vi "Analyse.vi"(8 "error in (no error)":errorcluster, 11 "ResultHandler JSON in":refnum<class "ResultHandler JSON.lvclass">) -> (0 "error out":errorcluster, 1 "ICallResult":refnum<class "ICallResult.lvclass">, 2 "Request ID":u64, 3 "ResultHandler JSON out":refnum<class "ResultHandler JSON.lvclass">)   [LabVIEW 2020, in "wamplv.lvlib" / "ResultHandler JSON.lvclass"]
uses:
  ResultHandler JSON.lvclass
  ResultHandler JSON.lvclass/ResultHandler JSON.ctl
  <vilib>/Utility/error.llb/Error Cluster From Error Code.vi
  <vilib>/ErrorRing/Error Ring.xnode
  Error/ErrorHandler JSON/ErrorHandler JSON.lvclass
  SerialisedMessages/JSONMessage/WampMessage JSON.lvclass
  Call/CallResult JSON/CallResult JSON.lvclass
  Utils/Utils.lvclass
  Call/ICallResult/ICallResult.lvclass
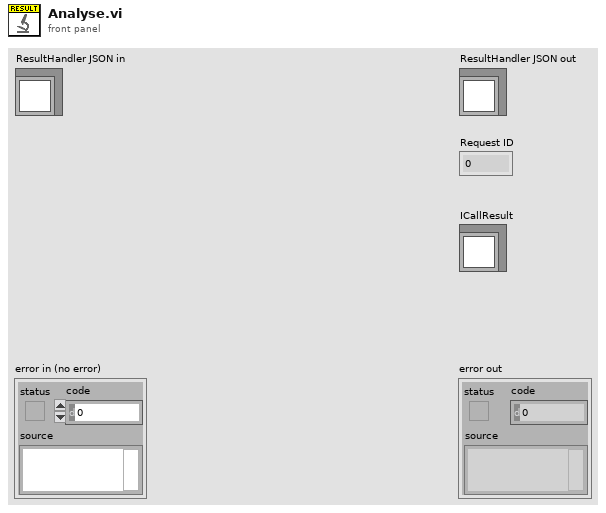
[diagram p1: front panel]
types:
  T1 = typedef "wamplv.lvlib/WAMP Message Codes.ctl" = enum8{"HELLO", "WELCOME", "CHALLENGE", "AUTHENTICATE", "ABORT", "GOODBYE", "ERROR", "PUBLISH", "PUBLISHED", "SUBSCRIBE", "SUBSCRIBED", "UNSUBSCRIBE", "UNSUBSCRIBED", "EVENT", "CALL", "RESULT", "REGISTER", "REGISTERED", "UNREGISTER", "UNREGISTERED", "INVOCATION", "YIELD"}
  T2 = typedef "wamplv.lvlib/Error (JSON).ctl" = cluster{"Request ID":u64, "Message type that caused error":T1, "Error/Abort details (JSON)":T3}
  T3 = typedef "wamplv.lvlib/Error or abort detail (JSON).ctl" = cluster{"Error URI":string, "Error Arguments":string, "Error ArgumentKw":string, "Error Details":string, "Associated LabVIEW Error":errorcluster}
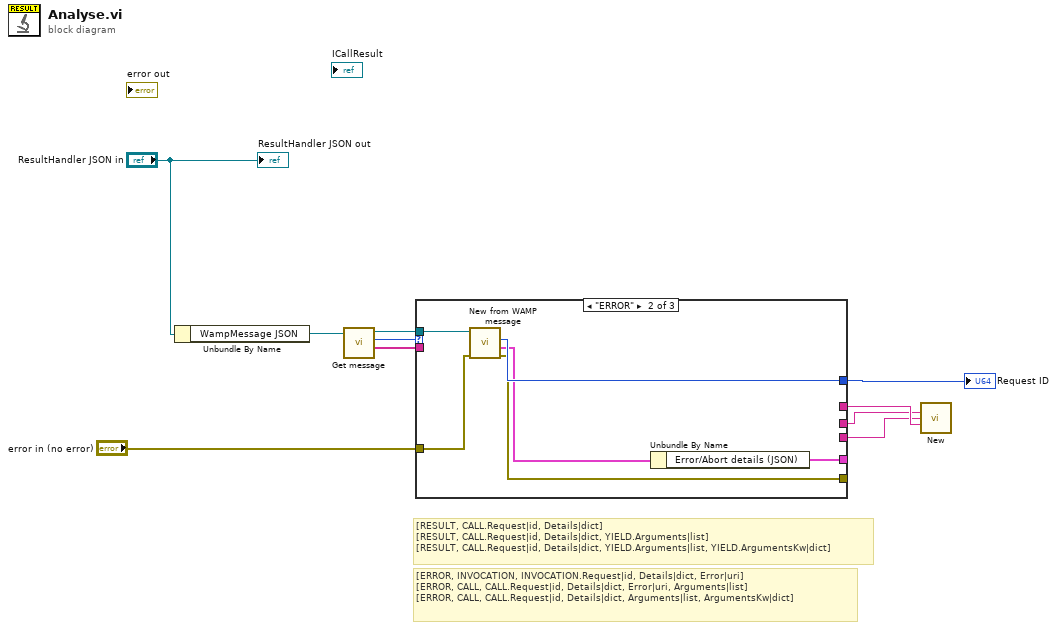
[diagram p0: block diagram]
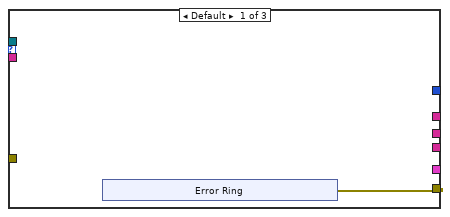
[diagram p2: hidden frame]
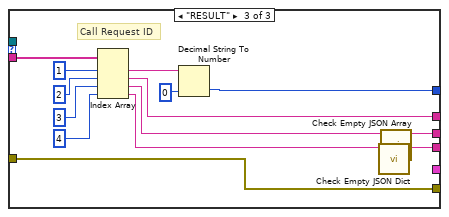
[diagram p3: hidden frame]
diagram:
  # "[RESULT, CALL.Request|id, Details|dict]\n[RESULT, CALL.Request|id, Details|dict, YIELD.Arguments|list]\n[RESULT, CALL.Request|id, Details|dict, YIELD.Arguments|list, YIELD.ArgumentsKw|dict]"
  # "[ERROR, INVOCATION, INVOCATION.Request|id, Details|dict, Error|uri]\n[ERROR, CALL, CALL.Request|id, Details|dict, Error|uri, Arguments|list]\n[ERROR, CALL, CALL.Request|id, Details|dict, Arguments|list, ArgumentsKw|dict]"
  n1 = Unbundle By Name("ResultHandler JSON in") -> ("WampMessage JSON"=w8:refnum<class "WampMessage JSON.lvclass">)
  n2 = call "Get message.vi"("JSONMessage in"=w8) -> ("<JSON>Elements"=w5:string[], "Message Type"=w7:T1, "JSONMessage out"=w6:refnum<class "WampMessage JSON.lvclass">)  [unwired: 8 in]
  n3 = case shown="\"ERROR\"" w7 {
    tunnel: [_ w18 w33] -> w4
    tunnel: [w11 w17 w32] -> _
    tunnel: [_ _ w22] -> w1
    tunnel: "error in (no error)" -> [_ w19 w32]
    tunnel: [_ w21 _] -> _
    tunnel: [_ _ w28] -> w3
    tunnel: [_ _ w24] -> w2
    tunnel: w6 -> [_ w20 _]
    tunnel: w5 -> [_ _ w27]
    frame Default {
      n4 = xnode "Error Ring"() -> ("error out"=w11:errorcluster)
    }
    frame "ERROR" {
      # "ERROR"
      n5 = call "New from WAMP message.vi"("error in (no error)"=w19, "wamplv.lvlib:JSONMessage.lvclass"=w20) -> ("error out"=w17:errorcluster, "Error data (JSON)"=w16:T2, "Request ID"=w18:u64)  [unwired: 6 in, 1 out]
      n6 = Unbundle By Name(w16) -> ("Error/Abort details (JSON)"=w21:T3)
    }
    frame "RESULT" {
      # "Call Request ID"
      # "RESULT"
      n7 = Index Array(array=w27, index #1=1 ("index"), index #2=2 ("index"), index #3=3 ("index"), index #4=4 ("index")) -> (element #1=w26:string, element #2=w28:string, element #3=w25:string, element #4=w23:string)
      n8 = Decimal String To Number(string=w26, default (0L)=u64 0) -> (number=w33:u64)  [unwired: 1 in, 1 out]
      n9 = call "Check Empty JSON Dict.vi"("JSON in"=w23) -> ("JSON out"=w22:string)  [unwired: 10 in]
      n10 = call "Check Empty JSON Array.vi"("JSON in"=w25) -> ("JSON out"=w24:string)  [unwired: 10 in]
    }
  }
  "Request ID" <- w4
  n11 = call "New.vi"("Arguments Payload"=w2, "ArgumentKw Payload"=w1, "Details"=w3) -> ()  [unwired: 12 in, 1 out]
  "ResultHandler JSON out" <- "ResultHandler JSON in"
